vi "DR200_control B_initialize.vi"(2 "B set (T)":dbl, 3 "Field Sweep Rate (T/min)":dbl min=-0.2 max=0.2, 4 "VISA Refnum in":refnum<visa-resource-name>) -> (1 "VISA Refnum out":refnum<visa-resource-name>)   [LabVIEW 2016]
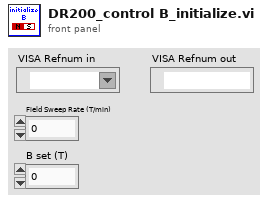
[diagram p1: front panel]
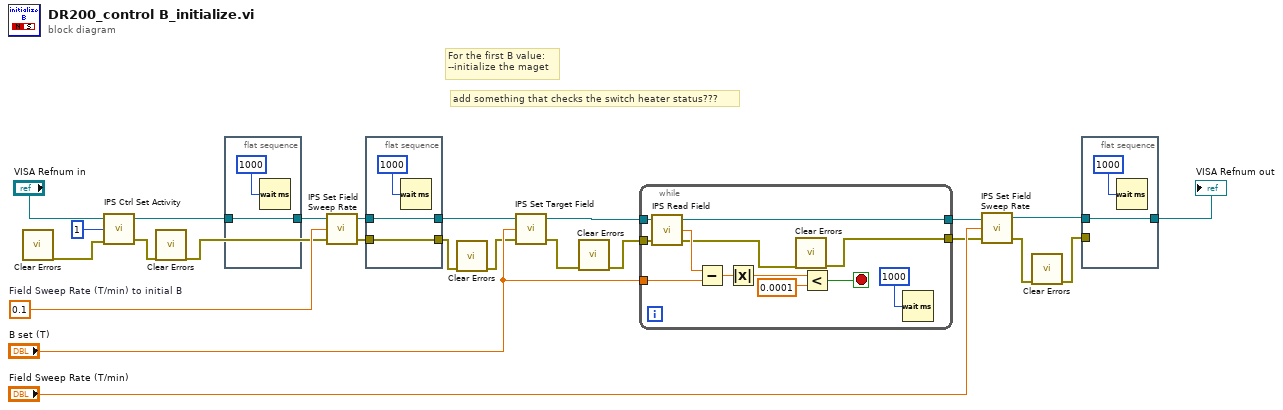
[diagram p0: block diagram]
diagram:
  w18 = 0.1  # Field Sweep Rate (T/min) to initial B
  # "add something that checks the switch heater status???"
  # "For the first B value:\n--initialize the maget"
  n1 = call <vilib>:"Clear Errors.vi"() -> ("error out"=w10:errorcluster)  [unwired: 6 in, 1 out]
  n2 = call "IPS Ctrl Set Activity.vi"("Error In"=w10, "Activity"=1, "VISA resource name (COM Port of Prologix Device)"="VISA Refnum in") -> ("Error Out"=w9:errorcluster, "VISA resource name (COM Port of Prologix Device) 2"=w12:refnum<visa-resource-name>)  [unwired: 1 out]
  n3 = call <vilib>:"Clear Errors.vi"("error in (no error)"=w9) -> ("error out"=w8:errorcluster)  [unwired: 5 in, 1 out]
  n4 = flat-sequence {
    tunnel: w12 -> [w26]
    tunnel: [w26] -> w13
    frame #0 {
      n5 = Wait (ms)(milliseconds to wait=u32 1000) -> ()  [unwired: 1 out]
    }
  }
  n6 = call "IPS Set Field Sweep Rate.vi"("Error In"=w8, "Field Sweep Rate (T/min)"=w18, "VISA resource name (COM Port of Prologix Device)"=w13) -> ("Error Out"=w11:errorcluster, "VISA resource name (COM Port of Prologix Device) 2"=w20:refnum<visa-resource-name>)  [unwired: 1 out]
  n7 = flat-sequence {
    tunnel: w20 -> [w29]
    tunnel: [w29] -> w19
    tunnel: w11 -> [w27]
    tunnel: [w27] -> w7
    frame #0 {
      n8 = Wait (ms)(milliseconds to wait=u32 1000) -> ()  [unwired: 1 out]
    }
  }
  n9 = call <vilib>:"Clear Errors.vi"("error in (no error)"=w7) -> ("error out"=w6:errorcluster)  [unwired: 5 in, 1 out]
  n10 = call "IPS Set Target Field.vi"("Error In"=w6, "Target Field (T)"="B set (T)", "VISA resource name"=w19) -> ("Error Out"=w4:errorcluster, "VISA resource name"=w24:refnum<visa-resource-name>)  [unwired: 1 out]
  n11 = call <vilib>:"Clear Errors.vi"("error in (no error)"=w4) -> ("error out"=w3:errorcluster)  [unwired: 5 in, 1 out]
  n12 = while {
    tunnel: "B set (T)" -> [w33]
    tunnel: w24 -> [w35]
    tunnel: [w34] -> w16
    tunnel: w3 -> [w32]
    tunnel: [w30] -> w5
    stop <- w38 stop-if-true
    n13 = call "IPS Read Field.vi"("Error In"=w32, "VISA resource name (COM Port of Prologix Device)"=w35) -> ("Error Out"=w31:errorcluster, "Field (T)"=w36:dbl, "VISA resource name (COM Port of Prologix Device) 2"=w34:refnum<visa-resource-name>)  [unwired: 1 in]
    n14 = Subtract(x=w36, y=w33) -> (x-y=w40:dbl)
    n15 = Absolute Value(x=w40) -> (abs(x)=w39:dbl)
    n16 = call <vilib>:"Clear Errors.vi"("error in (no error)"=w31) -> ("error out"=w30:errorcluster)  [unwired: 5 in, 1 out]
    n17 = Less?(x=w39, y=0.0001) -> (x < y?=w38:bool)
    n18 = Wait (ms)(milliseconds to wait=u32 1000) -> ()  [unwired: 1 out]
  }
  n19 = call "IPS Set Field Sweep Rate.vi"("Error In"=w5, "Field Sweep Rate (T/min)"="Field Sweep Rate (T/min)", "VISA resource name (COM Port of Prologix Device)"=w16) -> ("Error Out"=w2:errorcluster, "VISA resource name (COM Port of Prologix Device) 2"=w15:refnum<visa-resource-name>)  [unwired: 1 out]
  n20 = call <vilib>:"Clear Errors.vi"("error in (no error)"=w2) -> ("error out"=w1:errorcluster)  [unwired: 5 in, 1 out]
  n21 = flat-sequence {
    tunnel: w15 -> [w43]
    tunnel: [w43] -> w17
    tunnel: w1 -> [_]
    frame #0 {
      n22 = Wait (ms)(milliseconds to wait=u32 1000) -> ()  [unwired: 1 out]
    }
  }
  "VISA Refnum out" <- w17
